vi "Is Door Open.vi"(0 "Interface_object in":refnum<class "Timed Door.lvclass">, 5 "error in (no error)":errorcluster) -> (14 "Interface_object out":refnum<class "Timed Door.lvclass">, 16 "Is Door Open?":bool, 19 "error out":errorcluster)   [LabVIEW 2018, in "Timed Door.lvclass"]
uses:
  Timed Door.lvclass
  Timed Door.lvclass/Timed Door.ctl
  Get Door.vi
  Door/Door.lvclass
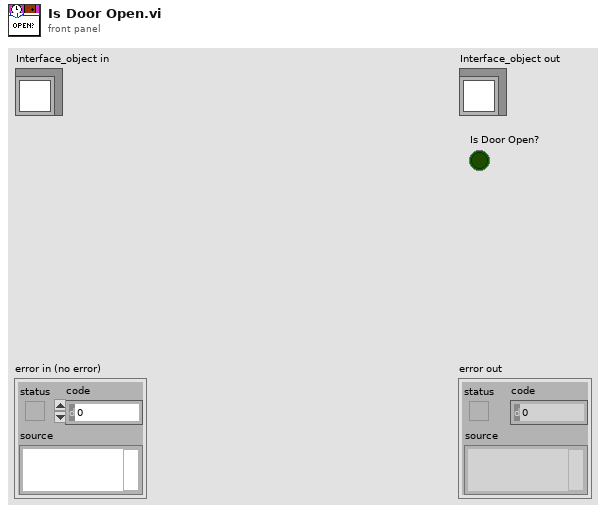
[diagram p1: front panel]
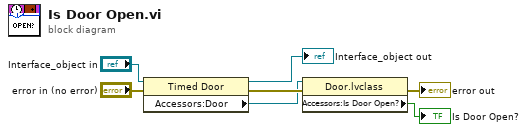
[diagram p0: block diagram]
diagram:
  n1 = property class="Timed Door"(reference="Interface_object in", error in="error in (no error)") -> (reference out=→"Interface_object out":refnum<class "Timed Door.lvclass">, error out=w7:errorcluster, "Accessors:Door"=w5:refnum<class "Door.lvclass">)
  n2 = property class="Door.lvclass"(reference=w5, error in=w7) -> (error out=→"error out":errorcluster, "Accessors:Is Door Open?"=→"Is Door Open?":bool)  [unwired: 1 out]
